vi "CAN_Demo_Template.vi"() -> ()   [LabVIEW 2014]
uses:
  TSMaster_API/All_Control/Typedef/Hardware Type.ctl
  Utilities/Typedef/Hardware_Subtype.ctl
  TSMaster_API/CAN_CANFD_Function/Typedef/TSCAN_CANFD_Configuration.ctl
  TSMaster_API/CAN_CANFD_Function/Typedef/TLibCANFD.ctl
panel:
  out "ACANMsgBuffer":T1(array[cluster])
  # "使用方法：\n1.创建TSMaster 工程，映射通道2，并开启接收Trace\n2.此demo 映射通道1\n3.通道1与通道2进行短接\n4.运行此demo 发送Fdata ,并接收Fdata"
  # "usage method:\n1. Create TSMaster project, map channel\n2, and enable receiving Trace. 2. This demo maps channel 1. \n3. Short circuit channel 1 to channel 2\n4. Run this demo sends and receives Fdata"
types:
  T1 = cluster{"FIdxChn":u8, "FProperties":u8, "FDLC":u8, "FReserved":u8, "FIdentifier":i32, "FTimeUS":u64, "Fdata":cluster{"初始化的数组[0]":u8, "初始化的数组[1]":u8, "初始化的数组[2]":u8, "初始化的数组[3]":u8, "初始化的数组[4]":u8, "初始化的数组[5]":u8, "初始化的数组[6]":u8, "初始化的数组[7]":u8, "初始化的数组[8]":u8, "初始化的数组[9]":u8, "初始化的数组[10]":u8, "初始化的数组[11]":u8, "初始化的数组[12]":u8, "初始化的数组[13]":u8, "初始化的数组[14]":u8, "初始化的数组[15]":u8, "初始化的数组[16]":u8, "初始化的数组[17]":u8, "初始化的数组[18]":u8, "初始化的数组[19]":u8, "初始化的数组[20]":u8, "初始化的数组[21]":u8, "初始化的数组[22]":u8, "初始化的数组[23]":u8, "初始化的数组[24]":u8, "初始化的数组[25]":u8, "初始化的数组[26]":u8, "初始化的数组[27]":u8, "初始化的数组[28]":u8, "初始化的数组[29]":u8, "初始化的数组[30]":u8, "初始化的数组[31]":u8, "初始化的数组[32]":u8, "初始化的数组[33]":u8, "初始化的数组[34]":u8, "初始化的数组[35]":u8, "初始化的数组[36]":u8, "初始化的数组[37]":u8, "初始化的数组[38]":u8, "初始化的数组[39]":u8, "初始化的数组[40]":u8, "初始化的数组[41]":u8, "初始化的数组[42]":u8, "初始化的数组[43]":u8, "初始化的数组[44]":u8, "初始化的数组[45]":u8, "初始化的数组[46]":u8, "初始化的数组[47]":u8, "初始化的数组[48]":u8, "初始化的数组[49]":u8, "初始化的数组[50]":u8, "初始化的数组[51]":u8, "初始化的数组[52]":u8, "初始化的数组[53]":u8, "初始化的数组[54]":u8, "初始化的数组[55]":u8, "初始化的数组[56]":u8, "初始化的数组[57]":u8, "初始化的数组[58]":u8, "初始化的数组[59]":u8, "初始化的数组[60]":u8, "初始化的数组[61]":u8, "初始化的数组[62]":u8, "初始化的数组[63]":u8}}[]
  T2 = typedef "TSCAN_CANFD_Configuration.ctl" = cluster{"Hardware Type":T3, "Hardware Subtype":T4, "AArbRateKbps":sgl, "AListenOnly":enum16{"Normal", "ListenOnly"}, "Int120Ohm":enum16{"Disable", "Enable"}, "EnableChannel":enum16{"Disable", "Enable"}, "AHwChannel":i32, "AAppChannel":i32, "ADataRateKbps":sgl, "AControllerType":i32, "AControllerMode":i32, "AldHW":i32}
  T3 = typedef "Hardware Type.ctl" = i32
  T4 = typedef "Hardware_Subtype.ctl" = enum16{"TS_UNKNOWN_DEVICE", "TSCAN_PRO", "TSCAN_Lite1", "TC1001", "TL1001", "TC1011", "TM5011", "TC1002", "TC1014", "TSCANFD2517", "TC1026", "TC1016", "TC1012", "TC1013", "TLog1002", "TC1034", "TC1018", "GW2116", "TC2115", "MP1013", "TC1113", "TC1114", "TP1013", "TC1017", "TP1018", "TF10XX", "TL1004_FD_4_LIN_2", "TE1051", "TP1051", "TP1034", "TTS9015", "TP1026", "TTS1026", "TTS1034", "TTS1018", "TL1011", "TTS1015_LiAuto", "TTS1013_LiAuto", "TTS1016Pro", "TC1054Pro", "TC1054", "TLog1038", "TO1013", "TC1034Pro", "TC1018Pro", "TC1038Pro", "TS_DEV_END"}
  T5 = typedef "TLibCANFD.ctl" = cluster{"AIdxchn":u8, "AId":i32, "AIsStd":u8, "BRS":enum16{"Close", "Open"}, "AIsData":u8, "ADLC":i32, "AIsFD":enum16{"Classic CAN Message", "FD CAN Message"}, "FDatas":cluster{"Initialize array[0]":u8, "Initialize array[1]":u8, "Initialize array[2]":u8, "Initialize array[3]":u8, "Initialize array[4]":u8, "Initialize array[5]":u8, "Initialize array[6]":u8, "Initialize array[7]":u8, "Initialize array[8]":u8, "Initialize array[9]":u8, "Initialize array[10]":u8, "Initialize array[11]":u8, "Initialize array[12]":u8, "Initialize array[13]":u8, "Initialize array[14]":u8, "Initialize array[15]":u8, "Initialize array[16]":u8, "Initialize array[17]":u8, "Initialize array[18]":u8, "Initialize array[19]":u8, "Initialize array[20]":u8, "Initialize array[21]":u8, "Initialize array[22]":u8, "Initialize array[23]":u8, "Initialize array[24]":u8, "Initialize array[25]":u8, "Initialize array[26]":u8, "Initialize array[27]":u8, "Initialize array[28]":u8, "Initialize array[29]":u8, "Initialize array[30]":u8, "Initialize array[31]":u8, "Initialize array[32]":u8, "Initialize array[33]":u8, "Initialize array[34]":u8, "Initialize array[35]":u8, "Initialize array[36]":u8, "Initialize array[37]":u8, "Initialize array[38]":u8, "Initialize array[39]":u8, "Initialize array[40]":u8, "Initialize array[41]":u8, "Initialize array[42]":u8, "Initialize array[43]":u8, "Initialize array[44]":u8, "Initialize array[45]":u8, "Initialize array[46]":u8, "Initialize array[47]":u8, "Initialize array[48]":u8, "Initialize array[49]":u8, "Initialize array[50]":u8, "Initialize array[51]":u8, "Initialize array[52]":u8, "Initialize array[53]":u8, "Initialize array[54]":u8, "Initialize array[55]":u8, "Initialize array[56]":u8, "Initialize array[57]":u8, "Initialize array[58]":u8, "Initialize array[59]":u8, "Initialize array[60]":u8, "Initialize array[61]":u8, "Initialize array[62]":u8, "Initialize array[63]":u8}}
  T6 = cluster{"数组[0]":u8, "数组[1]":u8, "数组[2]":u8, "数组[3]":u8, "数组[4]":u8, "数组[5]":u8, "数组[6]":u8, "数组[7]":u8, "数组[8]":u8, "数组[9]":u8, "数组[10]":u8, "数组[11]":u8, "数组[12]":u8, "数组[13]":u8, "数组[14]":u8, "数组[15]":u8, "数组[16]":u8, "数组[17]":u8, "数组[18]":u8, "数组[19]":u8, "数组[20]":u8, "数组[21]":u8, "数组[22]":u8, "数组[23]":u8, "数组[24]":u8, "数组[25]":u8, "数组[26]":u8, "数组[27]":u8, "数组[28]":u8, "数组[29]":u8, "数组[30]":u8, "数组[31]":u8, "数组[32]":u8, "数组[33]":u8, "数组[34]":u8, "数组[35]":u8, "数组[36]":u8, "数组[37]":u8, "数组[38]":u8, "数组[39]":u8, "数组[40]":u8, "数组[41]":u8, "数组[42]":u8, "数组[43]":u8, "数组[44]":u8, "数组[45]":u8, "数组[46]":u8, "数组[47]":u8, "数组[48]":u8, "数组[49]":u8, "数组[50]":u8, "数组[51]":u8, "数组[52]":u8, "数组[53]":u8, "数组[54]":u8, "数组[55]":u8, "数组[56]":u8, "数组[57]":u8, "数组[58]":u8, "数组[59]":u8, "数组[60]":u8, "数组[61]":u8, "数组[62]":u8, "数组[63]":u8}
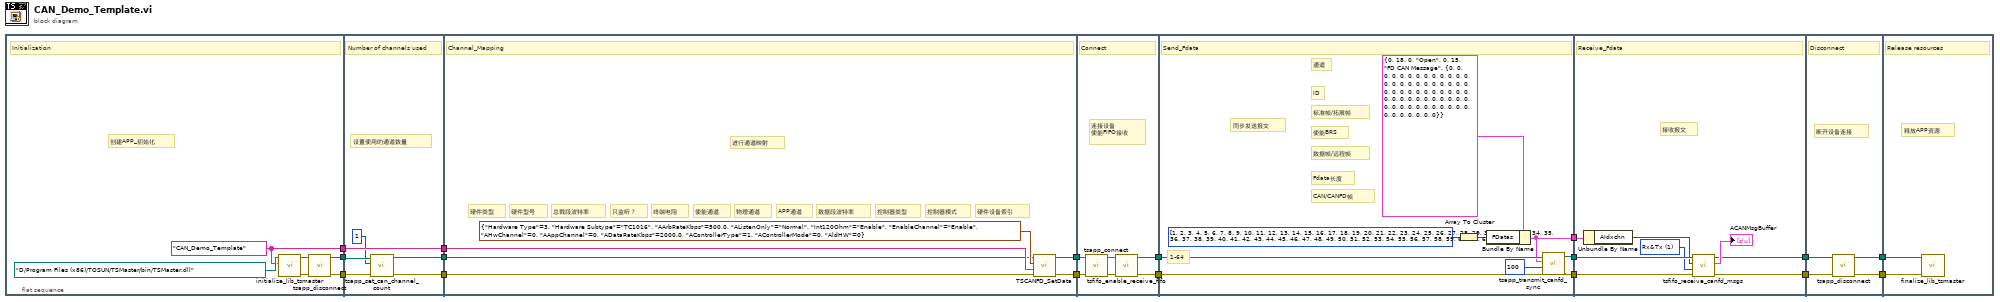
[diagram p0: block diagram]
diagram:
  n1 = flat-sequence {
    tunnel: [w20] -> w12
    tunnel: [w19] -> w11
    tunnel: [w18] -> w10
    tunnel: [w29] -> w13
    tunnel: w12 -> [w29]
    tunnel: w11 -> [w24]
    tunnel: w10 -> [w28]
    tunnel: [w26] -> w9
    tunnel: [w25] -> w8
    tunnel: [w34] -> w17
    tunnel: [w33] -> w16
    tunnel: w13 -> [w32]
    tunnel: w9 -> [w31]
    tunnel: w8 -> [w30]
    tunnel: w17 -> [w40]
    tunnel: w16 -> [w39]
    tunnel: [w37] -> w15
    tunnel: [w36] -> w14
    tunnel: w15 -> [w47]
    tunnel: w14 -> [w45]
    tunnel: [w44] -> w3
    tunnel: [w43] -> w2
    tunnel: [w46] -> w1
    tunnel: w3 -> [w58]
    tunnel: w2 -> [w57]
    tunnel: w1 -> [w56]
    tunnel: [w52] -> w7
    tunnel: [w51] -> w6
    tunnel: w7 -> [w62]
    tunnel: w6 -> [w61]
    tunnel: [w60] -> w5
    tunnel: [w59] -> w4
    tunnel: w5 -> [w64]
    tunnel: w4 -> [w63]
    frame #0 {
      w20 = "CAN_Demo_Template" ("AppName")
      # "创建APP_初始化"
      # "Initialization"
      n2 = call "initialize_lib_tsmaster.vi"("AppName"=w20, "Path input"=path "D:/Program Files (x86)/TOSUN/TSMaster/bin/TSMaster.dll") -> ("error output"=w22:errorcluster, "Path output"=w23:path)  [unwired: 8 in]
      n3 = call "tsapp_disconnect.vi"("error in (no error)"=w22, "Path"=w23) -> ("error output"=w19:errorcluster, "Path output"=w18:path)  [unwired: 7 in, 1 out]
    }
    frame #1 {
      # "设置使用的通道数量"
      # "Number of channels used"
      n4 = call "tsapp_set_can_channel_count.vi"("error in (no error)"=w24, "Aount"=1, "Path"=w28) -> ("error out"=w26:errorcluster, "Path output"=w25:path)  [unwired: 6 in, 1 out]
    }
    frame #2 {
      # "硬件设备索引"
      # "控制器模式"
      # "控制器类型"
      # "数据段波特率"
      # "APP通道"
      # "物理通道"
      # "使能通道"
      # "终端电阻"
      # "只监听？"
      # "总裁段波特率"
      # "硬件型号"
      # "硬件类型"
      # "进行通道映射"
      # "Channel_Mapping"
      n5 = call "TSCANFD_SetData.vi"("ERROR IN"=w31, "AppName"=w32, "CANFD Configuration"=T2 {"Hardware Type"=3, "Hardware Subtype"=enum."TC1016", "AArbRateKbps"=500.0, "AListenOnly"=enum."Normal", "Int120Ohm"=enum."Enable", "EnableChannel"=enum."Enable", "AHwChannel"=0, "AAppChannel"=0, "ADataRateKbps"=2000.0, "AControllerType"=1, "AControllerMode"=0, "AldHW"=0}, "PATH"=w30) -> ("ERROR OUT"=w33:errorcluster, "PATH OUT"=w34:path)  [unwired: 4 in, 2 out]
    }
    frame #3 {
      # "连接设备\n使能FIFO接收"
      # "Connect"
      n6 = call "tsapp_connect.vi"("error in (no error)"=w39, "Path"=w40) -> ("error out"=w41:errorcluster, "Path output"=w38:path)  [unwired: 7 in, 1 out]
      n7 = call "tsfifo_enable_receive_fifo.vi"("error in (no error)"=w41, "Path"=w38) -> ("error out"=w36:errorcluster, "Path output"=w37:path)  [unwired: 8 in]
    }
    frame #4 {
      # "CAN/CANFD帧"
      # "Fdata长度"
      # "数据帧/远程帧"
      # "使能BRS"
      # "标准帧/拓展帧"
      # "ID"
      # "通道"
      # "同步发送报文"
      # "1-64"
      # "Send_Fdata"
      n8 = Array To Cluster(array=u8[] [1, 2, 3, 4, 5, 6, 7, 8, 9, 10, 11, 12, 13, 14, 15, 16, 17, 18, 19, 20, 21, 22, 23, 24, 25, 26, 27, 28, 29, 30, 31, 32, 33, 34, 35, 36, 37, 38, 39, 40, 41, 42, 43, 44, 45, 46, 47, 48, 49, 50, 51, 52, 53, 54, 55, 56, 57, 58, 59, 60, 61, 62, 63, 64] ("数组")) -> (cluster=w48:T6)
      n9 = Bundle By Name(cluster=T5 {"AIdxchn"=0, "AId"=18, "AIsStd"=0, "BRS"=enum."Open", "AIsData"=0, "ADLC"=15, "AIsFD"=enum."FD CAN Message", "FDatas"={"Initialize array[0]"=0, "Initialize array[1]"=0, "Initialize array[2]"=0, "Initialize array[3]"=0, "Initialize array[4]"=0, "Initialize array[5]"=0, "Initialize array[6]"=0, "Initialize array[7]"=0, "Initialize array[8]"=0, "Initialize array[9]"=0, "Initialize array[10]"=0, "Initialize array[11]"=0, "Initialize array[12]"=0, "Initialize array[13]"=0, "Initialize array[14]"=0, "Initialize array[15]"=0, "Initialize array[16]"=0, "Initialize array[17]"=0, "Initialize array[18]"=0, "Initialize array[19]"=0, "Initialize array[20]"=0, "Initialize array[21]"=0, "Initialize array[22]"=0, "Initialize array[23]"=0, "Initialize array[24]"=0, "Initialize array[25]"=0, "Initialize array[26]"=0, "Initialize array[27]"=0, "Initialize array[28]"=0, "Initialize array[29]"=0, "Initialize array[30]"=0, "Initialize array[31]"=0, "Initialize array[32]"=0, "Initialize array[33]"=0, "Initialize array[34]"=0, "Initialize array[35]"=0, "Initialize array[36]"=0, "Initialize array[37]"=0, "Initialize array[38]"=0, "Initialize array[39]"=0, "Initialize array[40]"=0, "Initialize array[41]"=0, "Initialize array[42]"=0, "Initialize array[43]"=0, "Initialize array[44]"=0, "Initialize array[45]"=0, "Initialize array[46]"=0, "Initialize array[47]"=0, "Initialize array[48]"=0, "Initialize array[49]"=0, "Initialize array[50]"=0, "Initialize array[51]"=0, "Initialize array[52]"=0, "Initialize array[53]"=0, "Initialize array[54]"=0, "Initialize array[55]"=0, "Initialize array[56]"=0, "Initialize array[57]"=0, "Initialize array[58]"=0, "Initialize array[59]"=0, "Initialize array[60]"=0, "Initialize array[61]"=0, "Initialize array[62]"=0, "Initialize array[63]"=0}} ("TCANFD"), "FDatas"=w48) -> (w46:T5)
      n10 = call "tsapp_transmit_canfd_sync.vi"("error in (no error)"=w45, "ATimeoutMS"=100, "TCANFD"=w46, "Path"=w47) -> ("error out"=w43:errorcluster, "Path output"=w44:path)  [unwired: 5 in, 1 out]
    }
    frame #5 {
      w54 = u16 1 items=["Rx", "Rx&Tx"] ("Display message type")
      # "接收报文"
      # "Receive_Fdata"
      n11 = Unbundle By Name(w56) -> ("AIdxchn"=w55:u8)
      n12 = call "tsfifo_receive_canfd_msgs.vi"("error in (no error)"=w57, "Display message type"=w54, "AAPPChannel"=w55, "Path"=w58) -> ("error out"=w51:errorcluster, "ACANMsgBuffer"=→"ACANMsgBuffer":T1, "Path output"=w52:path)  [unwired: 3 in, 1 out]
    }
    frame #6 {
      # "断开设备连接"
      # "Disconnect"
      n13 = call "tsapp_disconnect.vi"("error in (no error)"=w61, "Path"=w62) -> ("error output"=w60:errorcluster, "Path output"=w59:path)  [unwired: 7 in, 1 out]
    }
    frame #7 {
      # "释放APP资源"
      # "Release resources"
      n14 = call "finalize_lib_tsmaster.vi"("error in (no error)"=w64, "Path"=w63) -> ()  [unwired: 8 in, 2 out]
    }
  }
